vi "test - case insensitive and space-safe.vi"(8 "error in (no error)":errorcluster, 11 "TestCase in":refnum<class "labview-config-library.lvclass">) -> (0 "error out":errorcluster, 3 "TestCase out":refnum<class "labview-config-library.lvclass">)   [LabVIEW 2017, in "labview-config-library.lvclass"]
uses:
  labview-config-library.lvclass
  <vilib>/addons/_JKI Toolkits/VI Tester/TestCase.llb/TestCase.lvclass
  INI-Static-Variable-Support/LabVIEW-Config/LabVIEW-Config.lvclass
  93deb637-a585-478e-9279-1a05f20924bf.vi
  2014b230-9b7a-4129-94a1-0f1e5270c384.vi
  346dd59e-d6f6-41a2-b483-808609c196fe.vi
  871779cb-2d6d-4066-bee5-0bd3fe6c7f1c.vi
  C:/Program Files (x86)/National Instruments/LabVIEW 2017/vi.lib/addons/_JKI Toolkits/VI Tester/TestCase.llb/TestCase.lvclass
panel:
  out "FileLogger Configuration-v1 2":T1={"Enable"=TRUE, "Limit"={"FileSize"=10000000, "FileNum"=2}, "Timestamp.Format"="%<%Y/%m/%d %H:%M:%S%3u>T", "AutoExit"=FALSE} {"Limit"."FileSize" format="%.0p"}
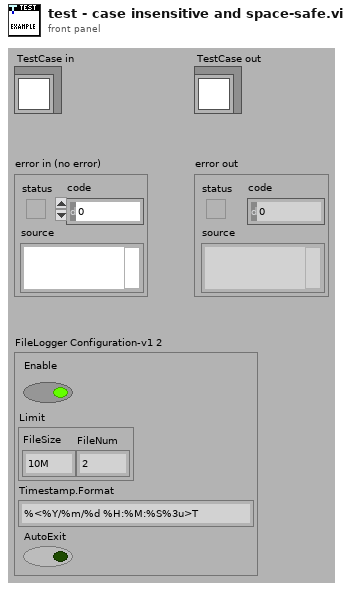
[diagram p1: front panel]
types:
  T1 = cluster{"Enable":bool, "Limit":cluster{"FileSize":i64, "FileNum":i32}, "Timestamp.Format":string, "AutoExit":bool}
  T2 = typedef "LabVIEW-Config.lvlib/LabVIEW-Config.lvclass/Config.ctl" = cluster{"Path":path, "Lines":string[], "Tokens":T3[], "Modified?":bool, "Cache":cluster{"Valid?":bool, "Key Information":T4[]}}
  T3 = typedef "LabVIEW-Config.lvlib/LabVIEW-Config.lvclass/LineToken.ctl" = enum8{"comment", "section", "key", "more"}
  T4 = typedef "LabVIEW-Config.lvlib/LabVIEW-Config.lvclass/KeyInfo.ctl" = cluster{"Key Indexes":cluster{"Indexes":i32[]}[], "Session Found?":bool, "Key found?":bool, "Session Index":i32}
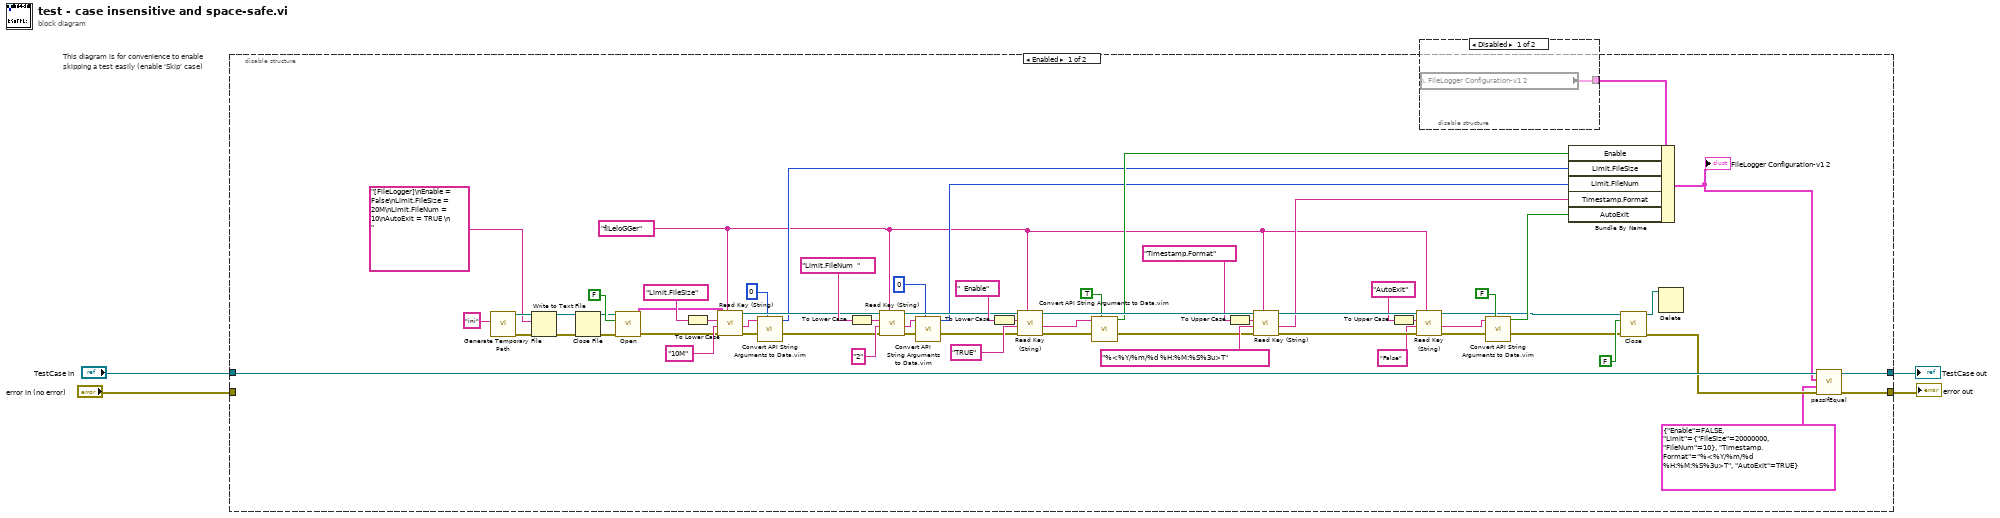
[diagram p0: block diagram]
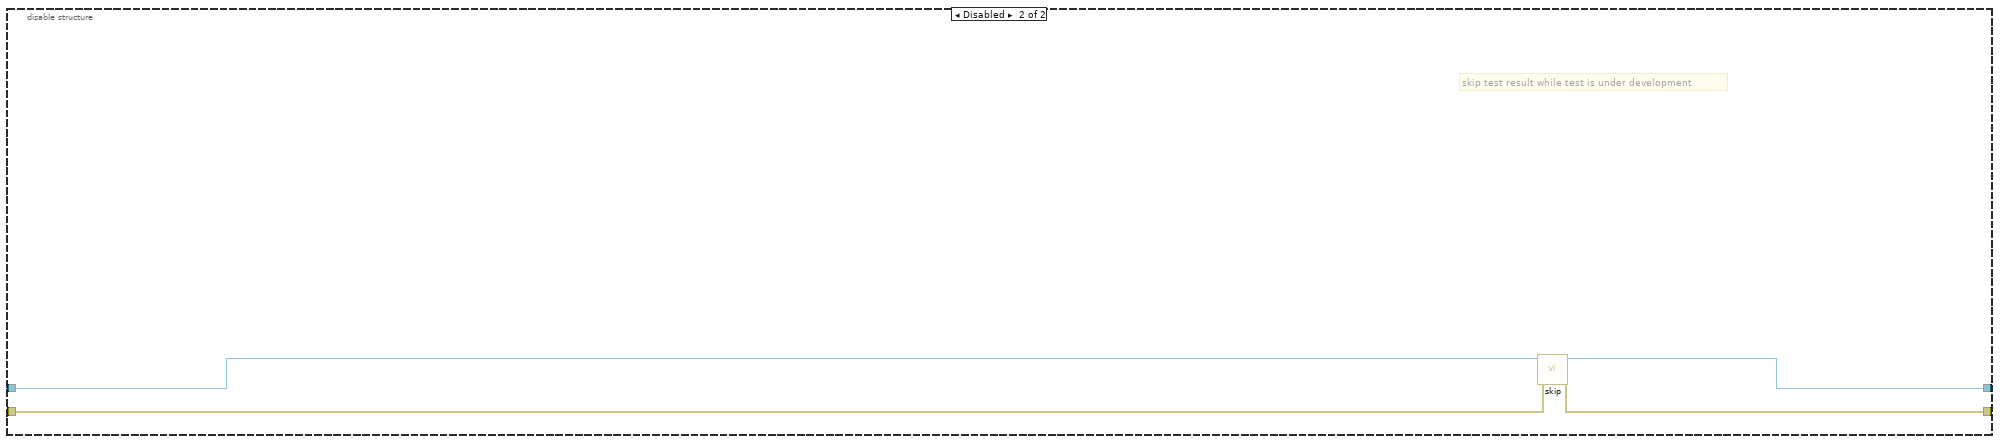
[diagram p3: hidden frame]
diagram:
  n1 = disable-structure "This diagram is for convenience to enable skipping a test easily (enable 'Skip' case)" shown="Enabled" {
    disable-tunnel: "TestCase in" -> [w67 w72]
    disable-tunnel: [w66 w70] -> w1
    disable-tunnel: [w65 w71] -> w3
    disable-tunnel: "error in (no error)" -> [_ w69]
    frame Enabled {
      w6 = "fiLeloGGer" ("Section Name")
      # "Create temporary ini file"
      n2 = call <vilib>:"Generate Temporary File Path.vi"("Temporary File Extension (tmp)"="ini") -> ("error out"=w62:errorcluster, "Unique Temporary File Path"=w59:path)  [unwired: 9 in]
      n3 = Write to Text File(file (use dialog)=w59, text="[FileLogger]\nEnable = False\nLimit.FileSize = 20M\nLimit.FileNum = 10\nAutoExit = TRUE \n ", error in=w62) -> (refnum out=w58:refnum<file>, error out=w60:errorcluster)  [unwired: 1 in, 1 out]
      n4 = Close File(refnum=w58, error in=w60) -> (path=w54:path, error out=w55:errorcluster)
      n5 = call "Open.vi"("error in (no error)"=w55, "Create if not exists? (T)"=FALSE, "Path"=w54) -> ("error out"=w14:errorcluster, "Config"=w15:T2)  [unwired: 5 in, 2 out]
      n6 = To Lower Case(string="Limit.FileSize" ("Key Name")) -> (all lower case string=w8:string)
      n7 = call "Read Key (String).vi"("Section Name"=w6, "error in (no error)"=w14, "Default"="10M", "Key Name"=w8, "Config in"=w15) -> ("error out"=w40:errorcluster, "Value"=w27:string, "Config out"=w39:refnum<class "LabVIEW-Config.lvclass">)  [unwired: 3 in, 1 out]
      n8 = call "Convert API String Arguments to Data.vim"("Type"=i64 0 ("Limit.FileSize"), "error in (no error)"=w40, "String"=w27) -> ("error"=w29:errorcluster, "Data"=w18:i64)  [unwired: 5 in]
      n9 = To Lower Case(string="Limit.FileNum  " ("Key Name")) -> (all lower case string=w9:string)
      n10 = call "Read Key (String).vi"("Section Name"=w6, "error in (no error)"=w29, "Default"="2", "Key Name"=w9, "Config in"=w39) -> ("error out"=w37:errorcluster, "Value"=w26:string, "Config out"=w38:refnum<class "LabVIEW-Config.lvclass">)  [unwired: 3 in, 1 out]
      n11 = call "Convert API String Arguments to Data.vim"("Type"=0 ("Limit.FileNum"), "error in (no error)"=w37, "String"=w26) -> ("error"=w30:errorcluster, "Data"=w16:i32)  [unwired: 5 in]
      n12 = To Lower Case(string="  Enable" ("Key Name")) -> (all lower case string=w7:string)
      n13 = call "Read Key (String).vi"("Section Name"=w6, "error in (no error)"=w30, "Default"="TRUE", "Key Name"=w7, "Config in"=w38) -> ("error out"=w46:errorcluster, "Value"=w25:string, "Config out"=w47:refnum<class "LabVIEW-Config.lvclass">)  [unwired: 3 in, 1 out]
      n14 = call "Convert API String Arguments to Data.vim"("Type"=TRUE, "error in (no error)"=w46, "String"=w25) -> ("error"=w28:errorcluster, "Data"=w22:bool)  [unwired: 5 in]
      n15 = To Upper Case(1:"Timestamp.Format" ("Key Name")) -> (0:w11:string)
      n16 = call "Read Key (String).vi"("Section Name"=w6, "error in (no error)"=w28, "Default"="%<%Y/%m/%d %H:%M:%S%3u>T", "Key Name"=w11, "Config in"=w47) -> ("error out"=w49:errorcluster, "Value"=w36:string, "Config out"=w50:refnum<class "LabVIEW-Config.lvclass">)  [unwired: 3 in, 1 out]
      n17 = To Upper Case(1:"AutoExit" ("Key Name")) -> (0:w10:string)
      n18 = call "Read Key (String).vi"("Section Name"=w6, "error in (no error)"=w49, "Default"="False", "Key Name"=w10, "Config in"=w50) -> ("error out"=w51:errorcluster, "Value"=w24:string, "Config out"=w5:refnum<class "LabVIEW-Config.lvclass">)  [unwired: 3 in, 1 out]
      n19 = disable-structure "Diagram Disable Structure" shown="Disabled" {
        disable-tunnel: [w68 _] -> w43
        frame Disabled {
          n20 = local read "FileLogger Configuration-v1 2"() -> (w68:T1)
        }
        frame Enabled {
        }
      }
      n21 = call "Convert API String Arguments to Data.vim"("Type"=FALSE, "error in (no error)"=w51, "String"=w24) -> ("error"=w13:errorcluster, "Data"=w20:bool)  [unwired: 5 in]
      n22 = Bundle By Name(cluster=w43, "Enable"=w22, "Limit.FileSize"=w18, "Limit.FileNum"=w16, "Timestamp.Format"=w36, "AutoExit"=w20) -> (w12:T1)
      "FileLogger Configuration-v1 2" <- w12
      n23 = call "Close.vi"("error in (no error)"=w13, "Write if modified? (T)"=FALSE, "Config"=w5) -> ("error out"=w53:errorcluster, "Path"=w56:path)  [unwired: 7 in]
      n24 = Delete(path (use dialog)=w56) -> ()  [unwired: 4 in, 3 out]
      n25 = call-dynamic "passIfEqual.vi"("error in (no error)"=w53, "y"=T1 {"Enable"=FALSE, "Limit"={"FileSize"=20000000, "FileNum"=10}, "Timestamp.Format"="%<%Y/%m/%d %H:%M:%S%3u>T", "AutoExit"=TRUE} ("FileLogger Configuration-v1"), "x"=w12, "TestCase in"=w67) -> ("error out"=w65:errorcluster, "TestCase out"=w66:refnum<class "labview-config-library.lvclass">)  [unwired: 6 in]
    }
    frame Disabled {
      # "skip test result while test is under development"
      n26 = call <vilib>:"skip.vi"("error in (no error)"=w69, "TestCase in"=w72) -> ("error out"=w71:errorcluster, "TestCase out"=w70:refnum<class "labview-config-library.lvclass">)  [unwired: 8 in]
    }
  }
  "error out" <- w3
  "TestCase out" <- w1
